vi "Do.vi"(8 "error in":errorcluster, 10 "Actor in":refnum<class "Actor.lvclass">, 11 "Sync Time MSG":refnum<class "Sync Time MSG.lvclass">) -> (0 "error out":errorcluster, 2 "Actor out":refnum<class "Actor.lvclass">)   [LabVIEW 2017, in "Controller.lvlib" / "Sync Time MSG.lvclass"]
doc: "(<B>Filename</B>: Actor Framework.lvlib:Message.lvclass:Do.vi)\n\nDefines what a message does when it is received by an actor. Generally, a message instructs an actor to invoke one of its methods. By default, this method does nothing. A child class must override it to define behavior. Create a child class by using the Actor Framework Message Maker dialog box."
uses:
  Sync Time MSG.lvclass
  <vilib>/ActorFramework/Actor/Actor.lvclass
  Sync Time MSG.lvclass/Sync Time MSG.ctl
  gController.lvclass
  C:/Program Files (x86)/National Instruments/LabVIEW 2017/vi.lib/MSR Consulting, LLC/General Reuse/SuperActor/SuperActor.lvclass
  C:/Program Files (x86)/National Instruments/LabVIEW 2017/vi.lib/ActorFramework/Actor/Actor.lvclass
  <vilib>/MSR Consulting, LLC/General Reuse/SuperActor/SuperActor.lvclass/SuperActor.ctl
  <vilib>/MSR Consulting, LLC/General Reuse/SuperActor/Read Log Session.vi
  <vilib>/MSR Consulting, LLC/General Reuse/Session APIs/_Session Fwk/Session - Root.lvclass
  <vilib>/MSR Consulting, LLC/General Reuse/Session APIs/Session Log/System Log.lvclass
  <vilib>/nisyscfg/nisyscfg.lvlib
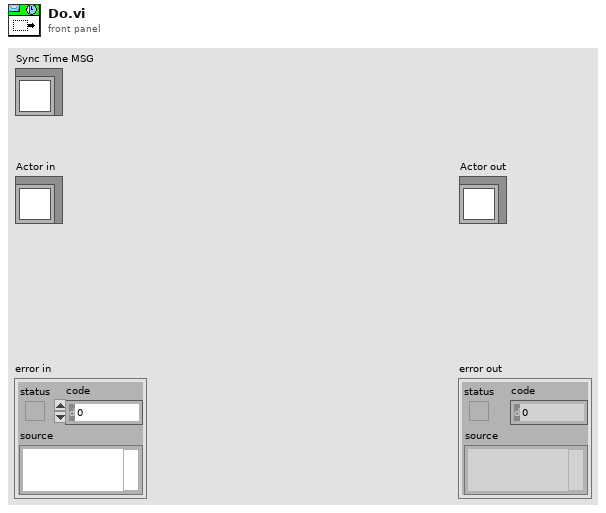
[diagram p1: front panel]
types:
  T1 = typedef "Session - Root.lvclass/Session Handle.ctl" = refnum<data-value>
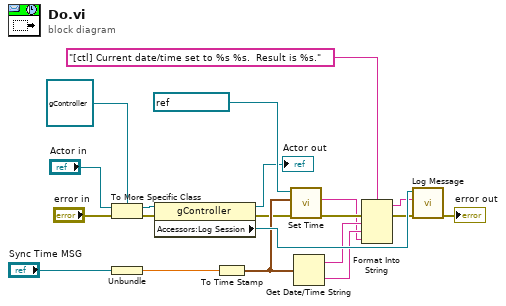
[diagram p0: block diagram]
diagram:
  n1 = To More Specific Class(target class=refnum<class "gController.lvclass"> refnum ("Controller.lvlib:gController"), reference="Actor in", error in="error in") -> (specific class reference=w17:refnum<class "gController.lvclass">, error out=w15:errorcluster)
  n2 = Unbundle("Sync Time MSG") -> (w13:dbl)
  n3 = property class="gController"(reference=w17, error in=w15) -> (reference out=→"Actor out":refnum<class "gController.lvclass">, error out=w4:errorcluster, "Accessors:Log Session"=w16:T1)
  n4 = To Time Stamp(1:w13) -> (0:w11:timestamp)
  n5 = call <vilib>:"Set Time.vi"("error in (no error)"=w4, "Time"=w11, "Session in (localhost)"=refnum<k21> "localhost") -> ("error out"=w5:errorcluster, "Detailed Result"=w3:string)  [unwired: 5 in, 2 out]
  n6 = Get Date/Time String(seconds (now)=w11) -> (date string=w9:string, time string=w8:string)  [unwired: 2 in]
  n7 = Format Into String(format string="[ctl] Current date/time set to %s %s.  Result is %s.", error in=w5, w9, w8, w3) -> (resulting string=w7:string, error out=w6:errorcluster)  [unwired: 1 in]
  n8 = call <vilib>:"Log Message.vi"("error in"=w6, "MSG In"=w7, "session in"=w16) -> ("error out"=→"error out":errorcluster)  [unwired: 7 in, 1 out]
